vi "Supply_Example.vi"() -> ()   [LabVIEW 2016]
uses:
  Source/Supply/Supply.lvlib
  Source/Supply/Typedefs/Supply Power Mode.ctl
  Source/Utilities/RDLUtilities.lvlib
  <instrlib>/niDCPower/nidcpower.llb/niDCPower Output Function.ctl
  Source/Supply/Typedefs/Custom Transient Response.ctl
  Source/Supply/Typedefs/Supply Configuration.ctl
  <instrlib>/niDCPower/nidcpower.llb/niDCPower Sense.ctl
  Source/Supply/Typedefs/Measurement Configuration.ctl
  Source/Supply/Typedefs/Measurement Results.ctl
panel:
  out "Status":string="Supply Switched OFF"
  in  "stop":bool
  out "Measurement Results":T1 {"Power (W)" format="%#_6p"; "Current (A)" format="%#_6p"; "Voltage (V)" format="%#_6p"}
  out "error out":errorcluster
  in  "Tab Control":enum32{"Configuration", "Measurement"}(tab)
  in  "Resource":refnum<k15>="4139"
  in  "Channels":string="0"
  in  "Supply Configuration":T2={"output function"=1006, "Voltage Level (V)"=3.0, "Current Level (A)"=0.001, "Voltage Limit (V)"=3.0, "Current Limit (A)"=1.0, "Transient Response Mode"=1038, "Custom Transient Config"={"Gain Bandwidth"=5000.0, "Compensation Frequency"=50000.0, "Pole Zero Ratio"=1.0}} {"Transient Response Mode" items=["Slow"=1041, "Normal"=1038, "Fast"=1039, "Custom"=1042]; "output function" items=["DC Voltage"=1006, "DC Current"=1007, "Pulse Voltage"=1049, "Pulse Current"=1050]}
  in  "Measurement Configuration":T5={"Measure When Mode"=1025, "Sense Mode"=1008, "Measurement Trigger Terminal"="PXI_Trig0", "Measurement Mode"=enum."Single Point", "Measurement Time (s)"=0.002} {"Measure When Mode" items=["Automatically after Source Complete"=1025, "On Demand"=1026, "On Measure Trigger"=1027]; "Sense Mode" items=["Local"=1008, "Remote"=1009]; "Measurement Time (s)" format="%#_13p"}
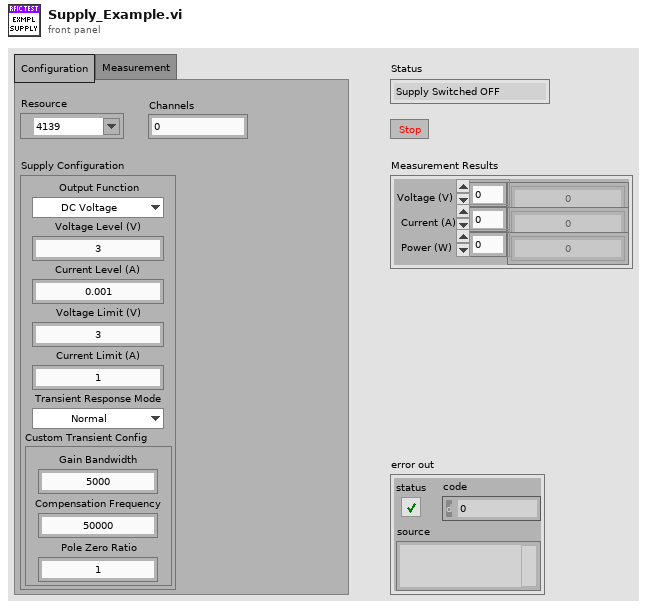
[diagram p1: front panel]
types:
  T1 = typedef "Supply.lvlib/Measurement Results.ctl" = cluster{"Voltage (V)":dbl[], "Current (A)":dbl[], "Power (W)":dbl[]}
  T2 = typedef "Supply.lvlib/Supply Configuration.ctl" = cluster{"output function":T3, "Voltage Level (V)":dbl, "Current Level (A)":dbl, "Voltage Limit (V)":dbl, "Current Limit (A)":dbl, "Transient Response Mode":i32, "Custom Transient Config":T4}
  T3 = typedef "niDCPower Output Function.ctl" = i32
  T4 = typedef "Supply.lvlib/Custom Transient Response.ctl" = cluster{"Gain Bandwidth":dbl, "Compensation Frequency":dbl, "Pole Zero Ratio":dbl}
  T5 = typedef "Supply.lvlib/Measurement Configuration.ctl" = cluster{"Measure When Mode":i32, "Sense Mode":T6, "Measurement Trigger Terminal":string, "Measurement Mode":enum16{"Single Point", "Record"}, "Measurement Time (s)":dbl}
  T6 = typedef "niDCPower Sense.ctl" = i32
  T7 = typedef "Supply.lvlib/Supply Power Mode.ctl" = enum16{"Power On", "Power Off"}
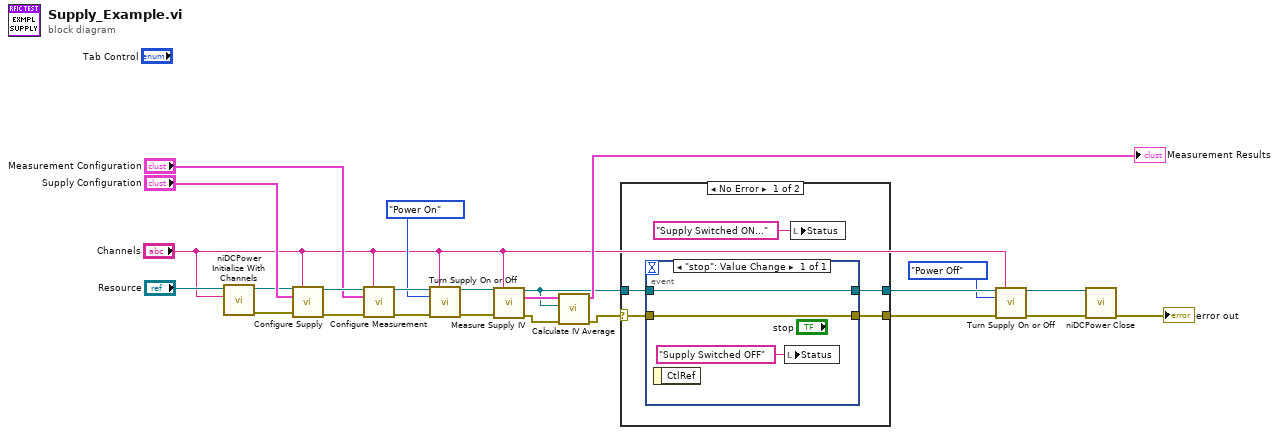
[diagram p0: block diagram]
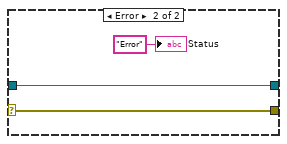
[diagram p2: hidden frame]
diagram:
  n1 = call <instrlib>:"niDCPower Initialize With Channels.vi"("channels"="Channels", "resource name"="Resource") -> ("error out"=w21:errorcluster, "instrument handle out"=w22:refnum<k15>)  [unwired: 8 in]
  n2 = call "Configure Supply.vi"("Supply Handle in"=w22, "Channel Name(s)"="Channels", "Supply Configuration"="Supply Configuration", "error in (no error)"=w21) -> ("Supply Handle out"=w20:refnum<k15>, "error out"=w19:errorcluster)  [unwired: 10 in]
  n3 = call "Configure Measurement.vi"("Supply Handle in"=w20, "Channel Name(s)"="Channels", "Measurement Configuration"="Measurement Configuration", "error in (no error)"=w19) -> ("Supply Handle out"=w17:refnum<k15>, "error out"=w14:errorcluster)  [unwired: 10 in]
  n4 = call "Turn Supply On or Off.vi"("Supply Handle in"=w17, "Channel Name(s)"="Channels", "Power Mode"=Supply_Power_Mode."Power On", "error in (no error)"=w14) -> ("Supply Handle out"=w15:refnum<k15>, "error out"=w13:errorcluster)  [unwired: 10 in]
  n5 = call "Measure Supply IV.vi"("Supply Handle in"=w15, "Channel Name(s)"="Channels", "error in (no error)"=w13) -> ("Supply Handle out"=w9:refnum<k15>, "Measurement Results"=w12:T1, "error out"=w10:errorcluster)  [unwired: 10 in]
  n6 = call "Calculate IV Average.vi"("error in (no error)"=w10, "Supply Line Handle in"=w9, "Supply Line Measurements Results in"=w12) -> ("error out"=w8:errorcluster, "Supply Line Measurements Results out"=→"Measurement Results":T1)  [unwired: 7 in]
  n7 = case shown="No Error" w8 {
    selector: w8 -> [w26 w35]
    tunnel: w9 -> [w29 w34]
    tunnel: [w28 w34] -> w3
    tunnel: [w27 w35] -> w7
    frame No Error {
      n8 = event shown="[0] \"stop\": Value Change" {
        selector: _ -> [_]
        dyn-events: _ -> [_]
        timeout: _ -> [_]
        tunnel: w26 -> [w31]
        tunnel: w29 -> [w32]
        tunnel: [w32] -> w28
        tunnel: [w31] -> w27
        event "stop": Value Change {
          n9 = event-data() -> ()  [unwired: 1 in, 1 out]
          n10 = local write "Status"("Supply Switched OFF" ("Status")) -> ()
        }
      }
      n11 = local write "Status"("Supply Switched ON..." ("Status")) -> ()
    }
    frame Error {
      "Status" <- "Error" ("Status")
    }
  }
  n12 = call "Turn Supply On or Off.vi"("Supply Handle in"=w3, "Channel Name(s)"="Channels", "Power Mode"=Supply_Power_Mode."Power Off", "error in (no error)"=w7) -> ("Supply Handle out"=w6:refnum<k15>, "error out"=w5:errorcluster)  [unwired: 10 in]
  n13 = call <instrlib>:"niDCPower Close.vi"("error in (no error)"=w5, "instrument handle"=w6) -> ("error out"=→"error out":errorcluster)  [unwired: 9 in]
